vi "Version 1_Batch Detect.vi"(7 "Address (A)":string="A", 8 "error in":errorcluster, 11 "VISA Session In":refnum<visa-resource-name>="Alicat") -> (0 "error out":errorcluster, 1 "Has Batch?":enum32{"Batch", "No Batch"}(radio), 3 "VISA Session Out":refnum<visa-resource-name>)   [LabVIEW 2020]
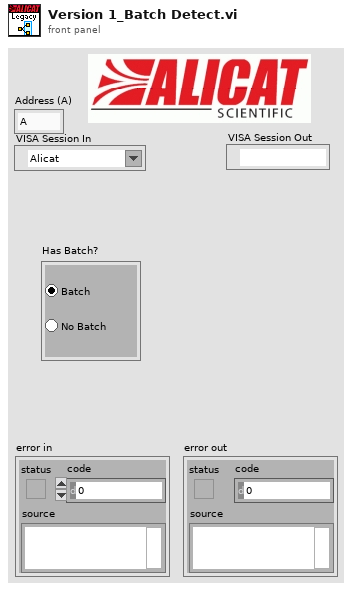
[diagram p1: front panel]
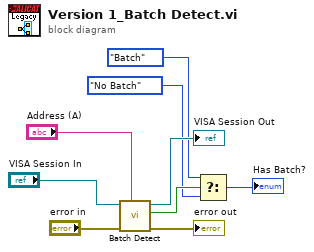
[diagram p0: block diagram]
diagram:
  n1 = call "Batch Detect.vi"("Unit ID (A)"="Address (A)", "error in"="error in", "VISA Session In"="VISA Session In") -> ("error out"=→"error out":errorcluster, "Batching available"=w3:bool, "VISA Session Out"=→"VISA Session Out":refnum<visa-resource-name>)  [unwired: 6 in]
  n2 = Select(t=enum32{"Batch", "No Batch"}."Batch" ("Has Batch?"), s=w3, f=enum32{"Batch", "No Batch"}."No Batch" ("Has Batch?")) -> (s? t:f=→"Has Batch?":enum32{"Batch", "No Batch"})
